vi "COMSelfTest.vi"(9 "error in (no error)":errorcluster caption="错误输入（无错误）") -> (1 "error out":errorcluster, 2 "COMOUT":refnum<visa-resource-name>)   [LabVIEW 2013]
uses:
  <vilib>/Instr/_visa.llb/VISA Configure Serial Port (Instr).vi
panel:
  out "Result":bool
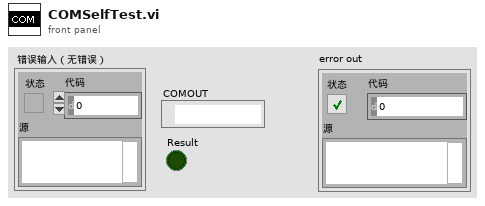
[diagram p1: front panel]
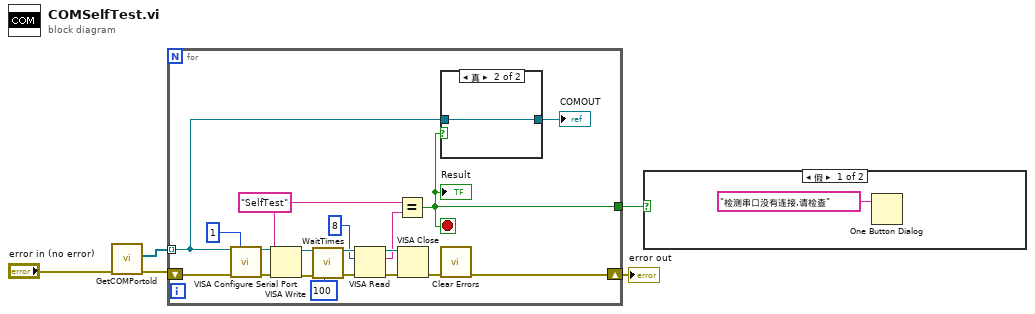
[diagram p0: block diagram]
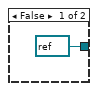
[diagram p3: hidden frame]
diagram:
  n1 = call "GetCOMPortold.vi"("error in"="error in (no error)") -> ("error out"=w1:errorcluster, "COMPort"=w5:refnum<visa-resource-name>[])  [unwired: 9 in]
  n2 = for {
    tunnel: w5 -> [w13] mode=indexing
    tunnel: [w11] -> w4
    shift-right: [w9] -> w3
    shift-left: w1 -> [w10]
    stop <- w11 stop-if-true
    w15 = "SelfTest" ("写入缓冲区")
    n3 = call-poly "VISA Configure Serial Port"("VISA resource name"=w13, "timeout (10sec)"=u32 1, "error in (no error)"=w10) -> ("VISA resource name out"=w23:refnum<visa-resource-name>, "error out"=w19:errorcluster)  [unwired: 11 in]
    n4 = VISA Write(VISA resource name=w23, write buffer=w15, error in (no error)=w19) -> (VISA resource name out=w22:refnum<visa-resource-name>, error out=w7:errorcluster)  [unwired: 1 out]
    n5 = call "WaitTimes.vi"("WaitTimes"=u32 100, "error in (no error)"=w7) -> ("error out"=w8:errorcluster)  [unwired: 9 in]
    n6 = VISA Read(VISA resource name=w22, byte count=u32 8 ("字节总数"), error in (no error)=w8) -> (VISA resource name out=w21:refnum<visa-resource-name>, read buffer=w14:string, error out=w20:errorcluster)  [unwired: 1 out]
    n7 = Equal?(x=w15, y=w14) -> (x = y?=w11:bool)
    "Result" <- w11
    n8 = VISA Close(VISA resource name=w21, error in (no error)=w20) -> (error out=w16:errorcluster)
    n9 = case shown="真" w11 {
      tunnel: w13 -> [_ w25]
      tunnel: [refnum<visa-resource-name> refnum ("VISA resource name") w25] -> w12
      frame False {
      }
      frame True {
      }
    }
    "COMOUT" <- w12
    n10 = call <vilib>:"Clear Errors.vi"("error in (no error)"=w16) -> ("error out"=w9:errorcluster)  [unwired: 6 in]
  }
  "error out" <- w3
  n11 = case shown="假" w4 {
    frame False {
      n12 = One Button Dialog(message="检测串口没有连接,请检查" ("消息")) -> ()  [unwired: 1 in, 1 out]
    }
    frame True {
    }
  }
